vi "Main.vi"(10 "DAQ Type":enum16{"Hardware", "Simulation"}(ring), 11 "Module Admin":refnum<class "Delacor_lib_QMH_Module Admin.lvclass">) -> ()   [LabVIEW 2021, in "DC PWS.lvlib"]
doc: "This template is based off of the Queued Message Handler design pattern and the Queued Message Handler project template that ships with LabVIEW.\n\nThe main difference is that the queue is private to this module and communication between modules is performed via Broadcast and Request events.\n\nRequest events are wrapped in public API methods and are handled in the Event Handling Loop (EHL) of this VI. Any module can register for Broadcast events sent by this module. The EHL generates messages based on user interface actions.\n\nThe Message Handling Loop (MHL) processes messages generated by the EHL, or by other messages. The messages are string values, so new messages can be added easily to the Message Cases case structure in the MHL. Each message cluster can also provide an optional value for Message Data, which is a variant that can be converted to whatever message-specific data is required.\n_____\nBased on DQMH Project Template 6.1.0.94."
uses:
  DC PWS.lvlib
  <vilib>/Delacor/Delacor QMH/Libraries/Module Admin_class/Delacor_lib_QMH_Module Admin.lvclass
  Class/BK-Precision/BK-Precision.lvclass
  C:/repository/common_ATE/Libraries/DC PWS/Class/Abstract/Abstract.lvclass
  Class/Abstract/Abstract.lvclass
  Module Data--cluster.ctl
  <vilib>/Delacor/Delacor QMH/Libraries/Message Queue_class/Delacor_lib_QMH_Message Queue.lvclass/Delacor_lib_QMH_Message Queue.ctl
  Stop Argument--cluster.ctl
  <vilib>/Delacor/Delacor QMH/Libraries/Module Admin_class/Delacor_lib_QMH_Module Admin.lvclass/Delacor_lib_QMH_Module Admin.ctl
  REQ Initialize Hardware Argument--cluster.ctl
  REQ Initialize Hardware (Reply Payload)--cluster.ctl
  REQ Config Current Limit Argument--cluster.ctl
  REQ Over Voltage Limit Argument--cluster.ctl
  REQ Configure Output Argument--cluster.ctl
  REQ Enable Output Argument--cluster.ctl
  REQ Measurement Argument--cluster.ctl
  REQ Measurement (Reply Payload)--cluster.ctl
  REQ Close Ref Argument--cluster.ctl
  <vilib>/Utility/miscctls.llb/LVPointTypeDef.ctl
  <vilib>/Delacor/Delacor QMH/Libraries/Message Queue_class/Delacor_lib_QMH_Enqueue Message (Single).vi
  <vilib>/Delacor/Delacor QMH/Libraries/Module Admin_class/Delacor_lib_QMH_Get External Launch.vi
  <vilib>/Utility/error.llb/Error Cluster From Error Code.vi
  <vilib>/ErrorRing/Error Ring.xnode
  <vilib>/Delacor/Delacor QMH/Libraries/Message Queue_class/Delacor_lib_QMH_Message Queue.lvclass
panel:
  out "error out":errorcluster
  out "Status":string
  in  "Simulate MHL Error":bool
  in  "Simulate EHL Error":bool
  # "Other QMH Modules communicate with this Module via its Public API (wrappers for its Request Events).\n\nThis Module communicates with other Modules via its Broadcast Events.\nAny module that wants to get these messages, just registers for this module's Broadcast events."
  # "This template is for the Delacor Modified Queued Message Handler design pattern.\n\nSee the block diagram for more information on how to use this template."
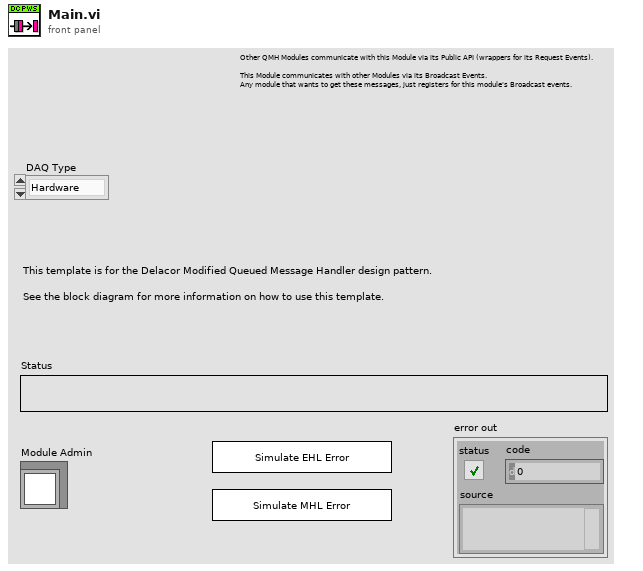
[diagram p1: front panel]
types:
  T1 = typedef "DC PWS.lvlib/Request Events--cluster.ctl" = cluster{"Stop Module":refnum<user-event>, "Show Panel":refnum<user-event>, "Hide Panel":refnum<user-event>, "Get Module Execution Status":refnum<user-event>, "Show Diagram":refnum<user-event>, "REQ Initialize Hardware":refnum<user-event>, "REQ Config Current Limit":refnum<user-event>, "REQ Over Voltage Limit":refnum<user-event>, "REQ Configure Output":refnum<user-event>, "REQ Enable Output":refnum<user-event>, "REQ Measurement":refnum<user-event>, "REQ Close Ref":refnum<user-event>}
  T2 = typedef "DC PWS.lvlib/Module Data--cluster.ctl" = cluster{"Status":string, "Abstract.lvclass":refnum<class "Abstract.lvclass">, "Connection Setting":cluster{"Connection Ref":variant, "Serial Configuration":cluster{"Baud Rate":u32}}}
  T3 = enum32{"invalid lock state", "Not Locked", "Locked (No Password)", "Password-protected"}
  T4 = typedef "DC PWS.lvlib/Stop Argument--cluster.ctl" = cluster{"Origin":string, "Exit via Stop Module Req?":bool, "Wait for Module to stop?":bool}
  T5 = typedef "DC PWS.lvlib/REQ Initialize Hardware Argument--cluster.ctl" = cluster{"Connection Setting":cluster{"Connection Ref":variant, "Serial Configuration":cluster{"Baud Rate":u32}}, "Wait Notifier":refnum<notifier>, "wait for reply":bool}
  T6 = typedef "DC PWS.lvlib/REQ Config Current Limit Argument--cluster.ctl" = cluster{"Current Limit Setting":cluster{"Address":dbl, "Current Limit":dbl}}
  T7 = typedef "DC PWS.lvlib/REQ Over Voltage Limit Argument--cluster.ctl" = cluster{"Over Voltage Setting":cluster{"Address":dbl, "Over Voltage Limit":dbl, "Protection Delay":dbl}}
  T8 = typedef "DC PWS.lvlib/REQ Configure Output Argument--cluster.ctl" = cluster{"Output Setting":cluster{"Address":dbl, "Voltage Level":dbl, "Enable Output":bool}}
  T9 = typedef "DC PWS.lvlib/REQ Enable Output Argument--cluster.ctl" = cluster{"Cluster":cluster{"Address":dbl, "Ouput":bool}}
  T10 = typedef "DC PWS.lvlib/REQ Measurement Argument--cluster.ctl" = cluster{"Wait Notifier":refnum<notifier>, "wait for reply":bool, "Meas Parameter":cluster{"Meas Command":enum16{"Voltage", "Current", "Power"}, "Address":dbl}}
  T11 = typedef "DC PWS.lvlib/REQ Close Ref Argument--cluster.ctl" = cluster{"Boolean":bool}
  T12 = typedef "LVPointTypeDef.ctl" = cluster{"Horizontal":i16, "Vertical":i16}
  T13 = enum32{"Invalid", "Standard", "Closed", "Hidden", "Minimized", "Maximized"}
  T14 = typedef "DC PWS.lvlib/REQ Initialize Hardware (Reply Payload)--cluster.ctl" = cluster{"Connect?":bool, "error":errorcluster}
  T15 = typedef "DC PWS.lvlib/REQ Measurement (Reply Payload)--cluster.ctl" = cluster{"error":errorcluster, "Value":dbl}
  T16 = cluster{"Connection Ref":variant, "Serial Configuration":cluster{"Baud Rate":u32}}
  T17 = cluster{"Address":dbl, "Over Voltage Limit":dbl, "Protection Delay":dbl}
  T18 = cluster{"Address":dbl, "Voltage Level":dbl, "Enable Output":bool}
  T19 = cluster{"Meas Command":enum16{"Voltage", "Current", "Power"}, "Address":dbl}
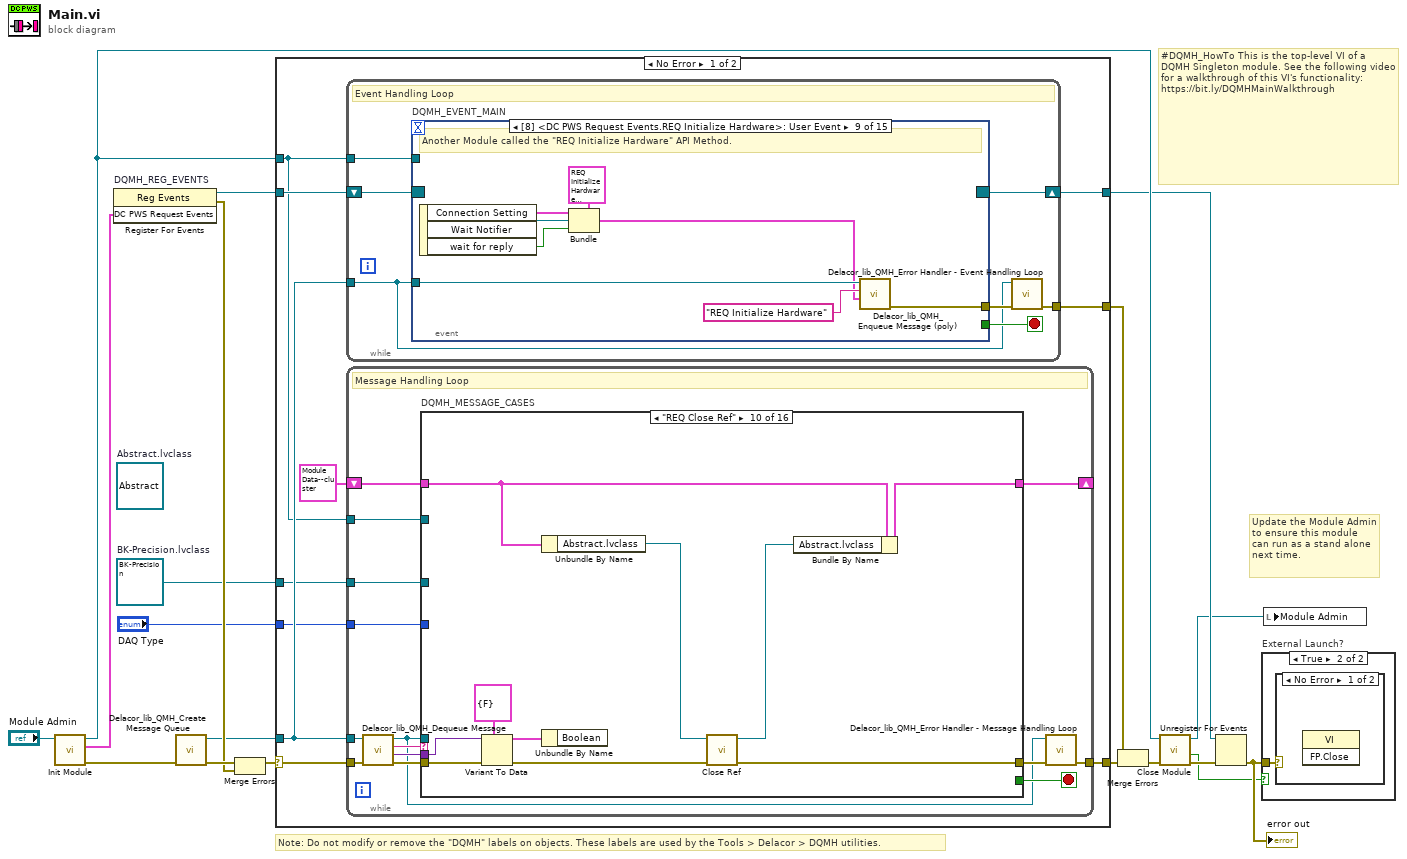
[diagram p0: block diagram]
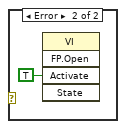
[diagram p3: hidden frame]
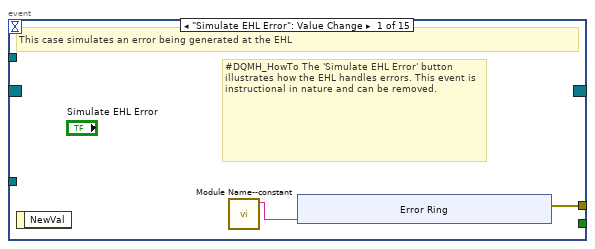
[diagram p4: hidden frame]
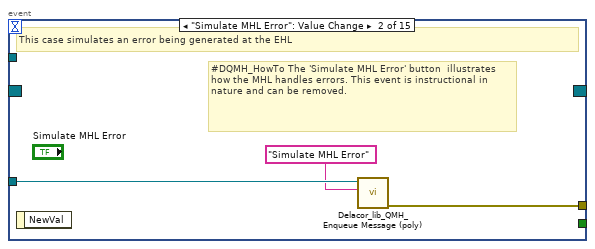
[diagram p5: hidden frame]
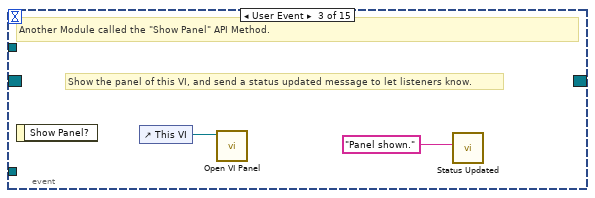
[diagram p6: hidden frame]
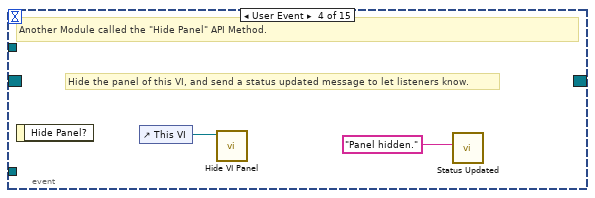
[diagram p7: hidden frame]
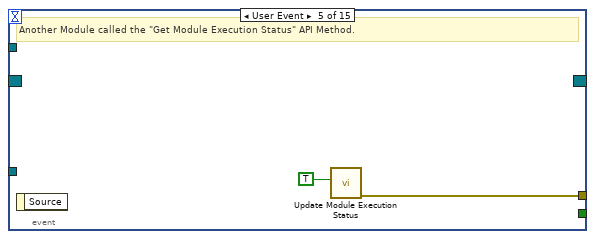
[diagram p8: hidden frame]
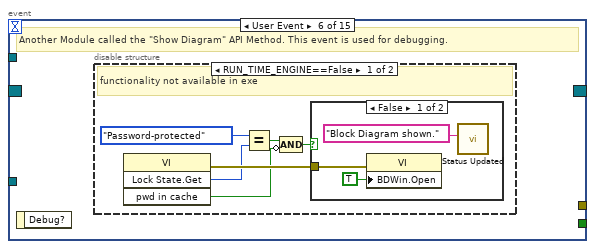
[diagram p9: hidden frame]
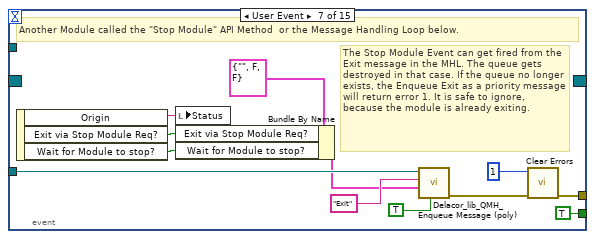
[diagram p12: hidden frame]
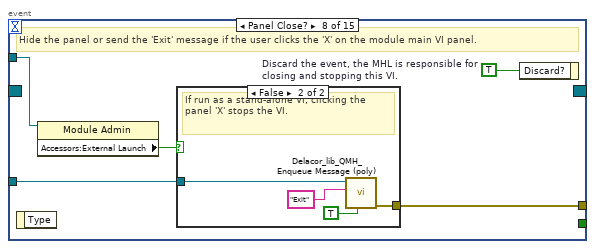
[diagram p13: hidden frame]
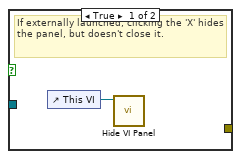
[diagram p14: hidden frame]
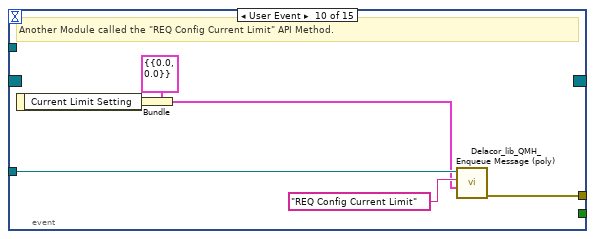
[diagram p15: hidden frame]
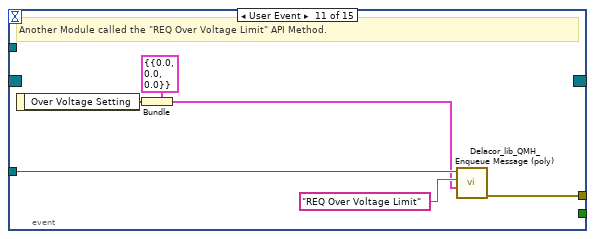
[diagram p16: hidden frame]
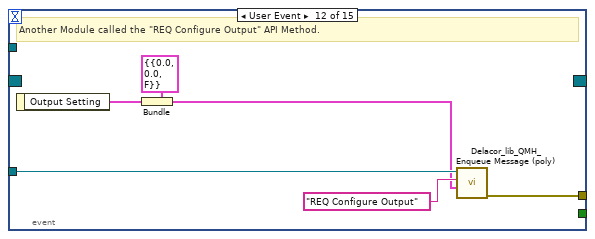
[diagram p17: hidden frame]
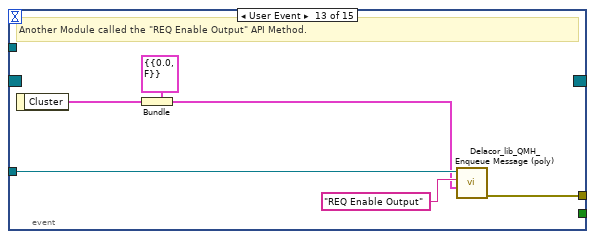
[diagram p18: hidden frame]
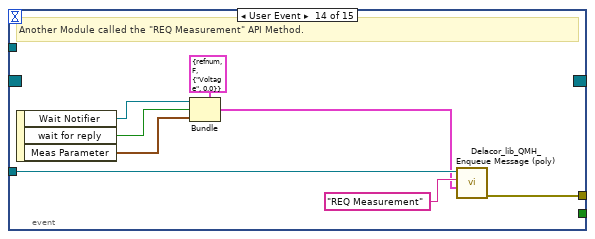
[diagram p19: hidden frame]
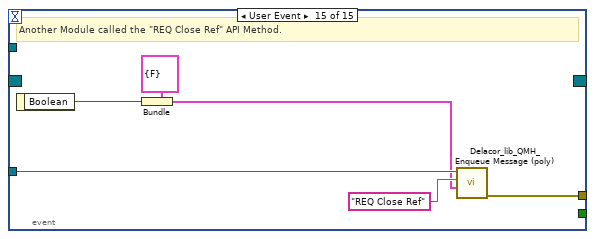
[diagram p20: hidden frame]
diagram:
  w2 = refnum<class "BK-Precision.lvclass"> refnum  # BK-Precision.lvclass
  (unwired) refnum<class "Abstract.lvclass"> refnum  # Abstract.lvclass
  # "#DQMH_HowTo This is the top-level VI of a DQMH Singleton module. See the following video for a walkthrough of this VI's functionality: https://bit.ly/DQMHMainWalkthrough"
  # "Note: Do not modify or remove the \"DQMH\" labels on objects. These labels are used by the Tools > Delacor > DQMH utilities."
  # "Update the Module Admin to ensure this module can run as a stand alone next time."
  n1 = call "Init Module.vi"("Singleton Module Admin in"="Module Admin") -> ("error out"=w18:errorcluster, "DC PWS Request Events"=w7:T1, "Singleton Module Admin out"=w10:refnum<class "Delacor_lib_QMH_Module Admin.lvclass">)  [unwired: 8 in]
  n2 = register-events "DQMH_REG_EVENTS"(w7) -> (reference out=w8:refnum<event-registration>, error out=w11:errorcluster)  [unwired: 2 in]
  n3 = call <vilib>:"Delacor_lib_QMH_Create Message Queue.vi"("error in"=w18) -> ("error out"=w13:errorcluster, "Message Queue"=w6:refnum<class "Delacor_lib_QMH_Message Queue.lvclass">)  [unwired: 9 in]
  n4 = Merge Errors(w13, w11) -> (w12:errorcluster)
  n5 = case shown="No Error" w12 {
    selector: w12 -> [w27 w339]
    tunnel: [w29 w338] -> w19
    tunnel: [w26 w344] -> w9
    tunnel: w8 -> [w24 w344]
    tunnel: w6 -> [w23 w337]
    tunnel: [w28 _] -> w16
    tunnel: w10 -> [w22 w340]
    tunnel: w2 -> [w21 _]
    tunnel: "DAQ Type" -> [w20 _]
    frame No Error {
      n6 = while {
        tunnel: w23 -> [w30]
        shift-right: [w33] -> w26
        shift-left: w24 -> [w34]
        tunnel: [w35] -> w28
        tunnel: w22 -> [w31]
        stop <- w32 stop-if-true
        # "Event Handling Loop"
        n7 = event "DQMH_EVENT_MAIN" shown="[8] <DC PWS Request Events.REQ Initialize Hardware>: User Event" {
          selector: w34 -> [_ _ _ _ _ _ _ _ _ _ _ _ _ _ _]
          dyn-events: [_ _ _ _ _ _ _ _ _ _ _ _ _ _ _] -> w33
          timeout: _ -> [_ _ _ _ _ _ _ _ _ _ _ _ _ _ _]
          tunnel: [_ _ _ _ _ _ TRUE ("Discard?") _ _ _ _ _ _ _ _] -> w32
          tunnel: w30 -> [_ w47 _ _ _ _ w71 w78 w93 w99 w105 w111 w117 w125 w131]
          tunnel: [w38 w48 _ _ w54 _ w74 w80 w86 w94 w100 w106 w112 w121 w126] -> w36
          tunnel: w31 -> [_ _ _ _ _ _ _ w77 _ _ _ _ _ _ _]
          event "Simulate EHL Error": Value Change {
            # "#DQMH_HowTo The 'Simulate EHL Error' button  illustrates how the EHL handles errors. This event is instructional in nature and can be removed."
            # "This case simulates an error being generated at the EHL"
            n8 = event-data() -> ()  [unwired: 1 in, 1 out]
            n9 = call "Module Name--constant.vi"() -> ("Module Name"=w37:string)  [unwired: 11 in]
            n10 = xnode "Error Ring"("parameter 0"=w37) -> ("error out"=w38:errorcluster)
          }
          event "Simulate MHL Error": Value Change {
            # "#DQMH_HowTo The 'Simulate MHL Error' button  illustrates how the MHL handles errors. This event is instructional in nature and can be removed."
            # "This case simulates an error being generated at the EHL"
            n11 = event-data() -> ()  [unwired: 1 in, 1 out]
            n12 = call-poly <vilib>:"Delacor_lib_QMH_Enqueue Message (poly).vi"("Message"="Simulate MHL Error", "Message Queue in"=w47) -> ("error out"=w48:errorcluster)  [unwired: 8 in, 1 out]
          }
          event User Event {
            # "Show the panel of this VI, and send a status updated message to let listeners know."
            # "Another Module called the \"Show Panel\" API Method."
            n13 = event-data() -> ()  [unwired: 1 in, 1 out]
            n14 = control-ref of="This VI"() -> (w50:refnum<vi>)
            n15 = call "Open VI Panel.vi"("VI"=w50) -> ()  [unwired: 10 in, 1 out]
            n16 = call "Status Updated.vi"("Status"="Panel shown." ("format string")) -> ()  [unwired: 10 in, 1 out]
          }
          event User Event {
            # "Hide the panel of this VI, and send a status updated message to let listeners know."
            # "Another Module called the \"Hide Panel\" API Method."
            n17 = event-data() -> ()  [unwired: 1 in, 1 out]
            n18 = control-ref of="This VI"() -> (w52:refnum<vi>)
            n19 = call "Hide VI Panel.vi"("VI"=w52) -> ()  [unwired: 10 in, 1 out]
            n20 = call "Status Updated.vi"("Status"="Panel hidden." ("format string")) -> ()  [unwired: 10 in, 1 out]
          }
          event User Event {
            # "Another Module called the \"Get Module Execution Status\" API Method."
            n21 = event-data() -> ()  [unwired: 1 in, 1 out]
            n22 = call "Update Module Execution Status.vi"("Running?"=TRUE) -> ("error out"=w54:errorcluster)  [unwired: 10 in]
          }
          event User Event {
            # "Another Module called the \"Show Diagram\" API Method. This event is used for debugging."
            n23 = event-data() -> ()  [unwired: 1 in, 1 out]
            n24 = disable-structure shown="RUN_TIME_ENGINE==False" {
              frame condition #0 (active) {
                # "functionality not available in exe"
                n25 = invoke class="VI" method="Lock State.Get"() -> (error out=w60:errorcluster, "Get Lock State"=w59:T3, "pwd in cache"=w56:bool)  [unwired: 4 in, 1 out]
                n26 = Equal?(x=T3."Password-protected", y=w59) -> (x = y?=w57:bool)
                n27 = Compound Arithmetic op=AND(w57, invert w56) -> (w55:bool)
                n28 = case shown="False" w55 {
                  tunnel: w60 -> [w63 _]
                  frame False {
                    n29 = property class="VI"(error in=w63, "BDWin.Open"=TRUE ("Block Diagram Window:Open")) -> ()  [unwired: 1 in, 2 out]
                    n30 = call "Status Updated.vi"("Status"="Block Diagram shown." ("format string")) -> ()  [unwired: 10 in, 1 out]
                  }
                  frame True {
                    # "Password-protected VI, and the password is not in the cache. Do not show the diagram."
                  }
                }
              }
              frame condition #1 {
              }
            }
          }
          event User Event {
            # "The Stop Module Event can get fired from the Exit message in the MHL. The queue gets destroyed in that case. If the queue no longer exists, the Enqueue Exit as a priority message will return error 1. It is safe to ignore, because the module is already exiting."
            # "Another Module called the \"Stop Module\" API Method  or the Message Handling Loop below."
            n31 = event-data() -> ("Origin"=w70:string, "Exit via Stop Module Req?"=w66:bool, "Wait for Module to stop?"=w65:bool)  [unwired: 1 in]
            n32 = local write "Status"(w70) -> ()
            n33 = Bundle By Name(cluster=T4 {"Origin"="", "Exit via Stop Module Req?"=FALSE, "Wait for Module to stop?"=FALSE} ("Stop Argument"), "Exit via Stop Module Req?"=w66, "Wait for Module to stop?"=w65) -> (w64:T4)
            n34 = call-poly <vilib>:"Delacor_lib_QMH_Enqueue Message (poly).vi"("Priority Message? (F)"=TRUE, "Message Data"=w64, "Message"="Exit", "Message Queue in"=w71) -> ("error out"=w75:errorcluster)  [unwired: 6 in, 1 out]
            n35 = call <vilib>:"Clear Errors.vi"("error in (no error)"=w75, "specific error code to clear (0: all)"=1) -> ("error out"=w74:errorcluster)  [unwired: 4 in, 1 out]
          }
          event Panel Close? {
            w79 = TRUE  # Discard the event, the MHL is responsible for closing and stopping this VI.
            # "Hide the panel or send the 'Exit' message if the user clicks the 'X' on the module main VI panel."
            n36 = event-data() -> ()  [unwired: 1 in, 1 out]
            n37 = property class="Module Admin"(reference=w77) -> ("Accessors:External Launch"=w76:bool)  [unwired: 1 in, 2 out]
            n38 = case shown="False" w76 {
              tunnel: w78 -> [_ w84]
              tunnel: [_ w85] -> w80
              frame True {
                # "If externally launched, clicking the 'X' hides the panel, but doesn't close it."
                n39 = control-ref of="This VI"() -> (w81:refnum<vi>)
                n40 = call "Hide VI Panel.vi"("VI"=w81) -> ()  [unwired: 10 in, 1 out]
              }
              frame False {
                # "If run as a stand-alone VI, clicking the panel 'X' stops the VI."
                n41 = call-poly <vilib>:"Delacor_lib_QMH_Enqueue Message (poly).vi"("Priority Message? (F)"=TRUE, "Message"="Exit", "Message Queue in"=w84) -> ("error out"=w85:errorcluster)  [unwired: 7 in, 1 out]
              }
            }
            n42 = event-data("Discard?"=w79) -> ()  [unwired: 1 in, 1 out]
          }
          event User Event {
            # "Another Module called the \"REQ Initialize Hardware\" API Method."
            n43 = event-data() -> ("Connection Setting"=w89:T16, "Wait Notifier"=w88:refnum<notifier>, "wait for reply"=w87:bool)  [unwired: 1 in]
            n44 = Bundle(cluster=T5 {"Connection Setting"={"Connection Ref"=variant, "Serial Configuration"={"Baud Rate"=9600}}, "Wait Notifier"=refnum, "wait for reply"=FALSE} ("REQ Initialize Hardware Argument"), "Connection Setting"=w89, "Wait Notifier"=w88, "wait for reply"=w87) -> (w90:T5)
            n45 = call-poly <vilib>:"Delacor_lib_QMH_Enqueue Message (poly).vi"("Message Data"=w90, "Message"="REQ Initialize Hardware", "Message Queue in"=w93) -> ("error out"=w86:errorcluster)  [unwired: 7 in, 1 out]
          }
          event User Event {
            # "Another Module called the \"REQ Config Current Limit\" API Method."
            n46 = event-data() -> ("Current Limit Setting"=w95:cluster{"Address":dbl, "Current Limit":dbl})  [unwired: 1 in]
            n47 = Bundle(cluster=T6 {"Current Limit Setting"={"Address"=0.0, "Current Limit"=0.0}} ("REQ Config Current Limit Argument"), "Current Limit Setting"=w95) -> (w96:T6)
            n48 = call-poly <vilib>:"Delacor_lib_QMH_Enqueue Message (poly).vi"("Message Data"=w96, "Message"="REQ Config Current Limit", "Message Queue in"=w99) -> ("error out"=w94:errorcluster)  [unwired: 7 in, 1 out]
          }
          event User Event {
            # "Another Module called the \"REQ Over Voltage Limit\" API Method."
            n49 = event-data() -> ("Over Voltage Setting"=w101:T17)  [unwired: 1 in]
            n50 = Bundle(cluster=T7 {"Over Voltage Setting"={"Address"=0.0, "Over Voltage Limit"=0.0, "Protection Delay"=0.0}} ("REQ Over Voltage Limit Argument"), "Over Voltage Setting"=w101) -> (w102:T7)
            n51 = call-poly <vilib>:"Delacor_lib_QMH_Enqueue Message (poly).vi"("Message Data"=w102, "Message"="REQ Over Voltage Limit", "Message Queue in"=w105) -> ("error out"=w100:errorcluster)  [unwired: 7 in, 1 out]
          }
          event User Event {
            # "Another Module called the \"REQ Configure Output\" API Method."
            n52 = event-data() -> ("Output Setting"=w107:T18)  [unwired: 1 in]
            n53 = Bundle(cluster=T8 {"Output Setting"={"Address"=0.0, "Voltage Level"=0.0, "Enable Output"=FALSE}} ("REQ Configure Output Argument"), "Output Setting"=w107) -> (w108:T8)
            n54 = call-poly <vilib>:"Delacor_lib_QMH_Enqueue Message (poly).vi"("Message Data"=w108, "Message"="REQ Configure Output", "Message Queue in"=w111) -> ("error out"=w106:errorcluster)  [unwired: 7 in, 1 out]
          }
          event User Event {
            # "Another Module called the \"REQ Enable Output\" API Method."
            n55 = event-data() -> ("Cluster"=w113:cluster{"Address":dbl, "Ouput":bool})  [unwired: 1 in]
            n56 = Bundle(cluster=T9 {"Cluster"={"Address"=0.0, "Ouput"=FALSE}} ("REQ Enable Output Argument"), "Cluster"=w113) -> (w114:T9)
            n57 = call-poly <vilib>:"Delacor_lib_QMH_Enqueue Message (poly).vi"("Message Data"=w114, "Message"="REQ Enable Output", "Message Queue in"=w117) -> ("error out"=w112:errorcluster)  [unwired: 7 in, 1 out]
          }
          event User Event {
            # "Another Module called the \"REQ Measurement\" API Method."
            n58 = event-data() -> ("Wait Notifier"=w120:refnum<notifier>, "wait for reply"=w119:bool, "Meas Parameter"=w118:T19)  [unwired: 1 in]
            n59 = Bundle(cluster=T10 {"Wait Notifier"=refnum, "wait for reply"=FALSE, "Meas Parameter"={"Meas Command"=enum."Voltage", "Address"=0.0}} ("REQ Measurement Argument"), "Wait Notifier"=w120, "wait for reply"=w119, "Meas Parameter"=w118) -> (w122:T10)
            n60 = call-poly <vilib>:"Delacor_lib_QMH_Enqueue Message (poly).vi"("Message Data"=w122, "Message"="REQ Measurement", "Message Queue in"=w125) -> ("error out"=w121:errorcluster)  [unwired: 7 in, 1 out]
          }
          event User Event {
            # "Another Module called the \"REQ Close Ref\" API Method."
            n61 = event-data() -> ("Boolean"=w127:bool)  [unwired: 1 in]
            n62 = Bundle(cluster=T11 {"Boolean"=FALSE} ("REQ Close Ref Argument"), "Boolean"=w127) -> (w128:T11)
            n63 = call-poly <vilib>:"Delacor_lib_QMH_Enqueue Message (poly).vi"("Message Data"=w128, "Message"="REQ Close Ref", "Message Queue in"=w131) -> ("error out"=w126:errorcluster)  [unwired: 7 in, 1 out]
          }
        }
        n64 = call-dynamic "Delacor_lib_QMH_Error Handler - Event Handling Loop.vi"("error in"=w36, "Message Queue in"=w30) -> ("dup error in"=w35:errorcluster)  [unwired: 8 in, 1 out]
      }
      n65 = while {
        tunnel: w23 -> [w136]
        shift-right: [w140] -> _
        shift-left: T2 {"Status"="", "Abstract.lvclass"=refnum, "Connection Setting"={"Connection Ref"=variant, "Serial Configuration"={"Baud Rate"=9600}}} ("Data Cluster") -> [w141]
        tunnel: w27 -> [w144]
        tunnel: [w142] -> w29
        tunnel: w22 -> [w134]
        tunnel: w21 -> [w133]
        tunnel: w20 -> [w132]
        stop <- w139 stop-if-true
        # "Message Handling Loop"
        n66 = call-dynamic "Delacor_lib_QMH_Dequeue Message.vi"("error in"=w144, "Message Queue in"=w136) -> ("error out"=w143:errorcluster, "Message Data"=w137:variant, "Message"=w138:string, "Message Queue out"=w135:refnum<class "Delacor_lib_QMH_Message Queue.lvclass">)  [unwired: 6 in]
        n67 = case "DQMH_MESSAGE_CASES" shown="\"REQ Close Ref\"" w138 {
          selector: w138 -> [_ _ _ _ _ _ _ _ _ _ _ _ _ _ _ w324]
          tunnel: w135 -> [_ _ _ _ _ _ _ _ w255 _ _ _ _ w289 w320 _]
          tunnel: w143 -> [w164 w168 w186 w199 w210 w221 w232 w248 w257 w269 w272 w274 w279 w296 w322 w326]
          tunnel: [w162 w168 w175 w194 w200 w216 w222 w234 w256 w264 w271 w274 w278 w292 w304 w327] -> w145
          tunnel: w141 -> [w153 w167 w170 w192 w204 w214 w226 w238 w254 w263 w270 w273 w276 w291 w311 w325]
          tunnel: [w152 w167 w177 w190 w202 w212 w224 w236 w254 w261 w270 w273 w276 w291 w308 w325] -> w140
          tunnel: [_ _ _ _ _ _ _ _ _ _ _ _ _ _ w319 _] -> w139
          tunnel: w137 -> [_ _ w185 w198 w209 w220 w231 w247 _ w268 _ _ _ w290 w318 _]
          tunnel: w134 -> [w154 _ _ _ _ _ _ _ _ _ _ _ _ w288 w313 _]
          tunnel: w133 -> [w146 _ _ _ _ _ _ _ _ _ _ _ _ _ _ _]
          tunnel: w132 -> [_ _ w172 _ _ _ _ _ _ _ _ _ _ _ _ _]
          frame "Initialize" {
            w148 = "Initial Message" ("Initial Message")
            # "Initialize - Any operation that needs to be done before the module can receive messages. Synchronize Caller Events.vi will inform Start Module.vi that the module has launched and is ready to receive messages. Module Did Init.vi will broadcast that the module initialized."
            n68 = call "Synchronize Caller Events.vi"("error in (no error)"=w164, "Singleton Module Admin in"=w154) -> ("error out"=w163:errorcluster, "Singleton Module Admin out"=w149:refnum<class "Delacor_lib_QMH_Module Admin.lvclass">)  [unwired: 8 in]
            n69 = property class="Module Admin"(reference=w149) -> ("Accessors:External Launch"=w158:bool)  [unwired: 1 in, 2 out]
            n70 = Select(t=T13."Hidden" ("State"), s=w158, f=T13."Standard" ("State")) -> (s? t:f=w155:T13)
            n71 = call "Module Name--constant.vi"() -> ("Module Name"=w161:string)  [unwired: 11 in]
            n72 = Bundle By Name(cluster=w153, "Status"=w148, "Abstract.lvclass"=w146) -> (w152:T2)
            n73 = property class="VI"("Front Panel.Title"=w161) -> (reference out=w160:refnum<vi>, error out=w166:errorcluster)  [unwired: 2 in]
            n74 = call "Module Name--constant.vi"() -> ("Module Name"=w150:string)  [unwired: 11 in]
            n75 = invoke class="VI" method="FP.Open"(reference=w160, error in=w166, "State"=w155) -> (reference out=w159:refnum<vi>, error out=w165:errorcluster)  [unwired: 2 in, 3 out]
            n76 = call "Module Did Init.vi"("error in (no error)"=w163, "Initialized?"=TRUE, "Origin"=w150) -> ("error out"=w162:errorcluster)  [unwired: 8 in]
            n77 = invoke class="VI" method="FP.Center"(reference=w159, error in=w165) -> ()  [unwired: 1 in, 3 out]
            n78 = property on="Pane" class="Pane"("Origin"=T12 {"Horizontal"=0, "Vertical"=0}) -> ()  [unwired: 2 in, 2 out]
            "Status" <- w148
          }
          frame "---Module Specific---" {
            # "Separator -- The following cases handle messages specific to this Module."
          }
          frame "REQ Initialize Hardware" {
            n79 = Variant To Data(error in=w186, type=T5 {"Connection Setting"={"Connection Ref"=variant, "Serial Configuration"={"Baud Rate"=9600}}, "Wait Notifier"=refnum, "wait for reply"=FALSE} ("REQ Initialize Hardware Argument"), Variant=w185) -> (data=w183:T5, error out=w178:errorcluster)
            n80 = Unbundle By Name(w183) -> ("Wait Notifier"=w182:refnum<notifier>, "wait for reply"=w181:bool, "Connection Setting"=w171:T16)
            n81 = Unbundle By Name(w170) -> ("Abstract.lvclass"=w169:refnum<class "Abstract.lvclass">)
            n82 = call-dynamic "Initialize Hardware.vi"("error in (no error)"=w178, "Connection Setting"=w171, "DAQ Type"=w172, "Abstract in"=w169) -> ("error out"=w175:errorcluster, "Abstract out"=w176:refnum<class "Abstract.lvclass">)  [unwired: 6 in]
            n83 = Unbundle By Name(w175) -> ("status"=w174:bool)
            n84 = Bundle By Name(cluster=w170, "Connection Setting"=w171, "Abstract.lvclass"=w176) -> (w177:T2)
            n85 = Not(x=w174) -> (.not. x?=w173:bool)
            n86 = Bundle By Name(cluster=T14 {"Connect?"=FALSE, "error"={"status"=FALSE, "code"=0, "source"=""}} ("REQ Initialize Hardware (Reply Payload)"), "Connect?"=w173) -> (w180:T14)
            n87 = case shown="True" w181 {
              tunnel: w182 -> [_ w188]
              tunnel: w180 -> [_ w187]
              frame False {
              }
              frame True {
                n88 = Send Notification(notification=w187, notifier=w188) -> ()  [unwired: 1 in, 2 out]
              }
            }
          }
          frame "REQ Config Current Limit" {
            n89 = Variant To Data(error in=w199, type=T6 {"Current Limit Setting"={"Address"=0.0, "Current Limit"=0.0}} ("REQ Config Current Limit Argument"), Variant=w198) -> (data=w196:T6, error out=w195:errorcluster)
            n90 = Unbundle By Name(w196) -> ("Current Limit Setting"=w193:cluster{"Address":dbl, "Current Limit":dbl})
            n91 = Unbundle By Name(w192) -> ("Abstract.lvclass"=w191:refnum<class "Abstract.lvclass">)
            n92 = call-dynamic "Configure Current Limit.vi"("error in (no error)"=w195, "Current Limit Setting"=w193, "Abstract in"=w191) -> ("error out"=w194:errorcluster, "Abstract out"=w189:refnum<class "Abstract.lvclass">)  [unwired: 7 in]
            n93 = Bundle By Name(cluster=w192, "Abstract.lvclass"=w189) -> (w190:T2)
          }
          frame "REQ Over Voltage Limit" {
            n94 = Variant To Data(error in=w210, type=T7 {"Over Voltage Setting"={"Address"=0.0, "Over Voltage Limit"=0.0, "Protection Delay"=0.0}} ("REQ Over Voltage Limit Argument"), Variant=w209) -> (data=w207:T7, error out=w206:errorcluster)
            n95 = Unbundle By Name(w207) -> ("Over Voltage Setting"=w205:T17)
            n96 = Unbundle By Name(w204) -> ("Abstract.lvclass"=w203:refnum<class "Abstract.lvclass">)
            n97 = call-dynamic "Configure Over Voltage Limit.vi"("error in (no error)"=w206, "Over Voltage Setting"=w205, "Abstract in"=w203) -> ("error out"=w200:errorcluster, "Abstract out"=w201:refnum<class "Abstract.lvclass">)  [unwired: 7 in]
            n98 = Bundle By Name(cluster=w204, "Abstract.lvclass"=w201) -> (w202:T2)
          }
          frame "REQ Configure Output" {
            n99 = Variant To Data(error in=w221, type=T8 {"Output Setting"={"Address"=0.0, "Voltage Level"=0.0, "Enable Output"=FALSE}} ("REQ Configure Output Argument"), Variant=w220) -> (data=w218:T8, error out=w217:errorcluster)
            n100 = Unbundle By Name(w218) -> ("Output Setting"=w215:T18)
            n101 = Unbundle By Name(w214) -> ("Abstract.lvclass"=w213:refnum<class "Abstract.lvclass">)
            n102 = call-dynamic "Configure Output.vi"("error in (no error)"=w217, "Output Setting"=w215, "Abstract in"=w213) -> ("error out"=w216:errorcluster, "Abstract out"=w211:refnum<class "Abstract.lvclass">)  [unwired: 7 in]
            n103 = Bundle By Name(cluster=w214, "Abstract.lvclass"=w211) -> (w212:T2)
          }
          frame "REQ Enable Output" {
            n104 = Variant To Data(error in=w232, type=T9 {"Cluster"={"Address"=0.0, "Ouput"=FALSE}} ("REQ Enable Output Argument"), Variant=w231) -> (data=w229:T9, error out=w228:errorcluster)
            n105 = Unbundle By Name(w229) -> ("Cluster"=w227:cluster{"Address":dbl, "Ouput":bool})
            n106 = Unbundle By Name(w226) -> ("Abstract.lvclass"=w225:refnum<class "Abstract.lvclass">)
            n107 = call-dynamic "Enable Output.vi"("error in (no error)"=w228, "Cluster"=w227, "Abstract in"=w225) -> ("error out"=w222:errorcluster, "Abstract out"=w223:refnum<class "Abstract.lvclass">)  [unwired: 7 in]
            n108 = Bundle By Name(cluster=w226, "Abstract.lvclass"=w223) -> (w224:T2)
          }
          frame "REQ Measurement" {
            n109 = Variant To Data(error in=w248, type=T10 {"Wait Notifier"=refnum, "wait for reply"=FALSE, "Meas Parameter"={"Meas Command"=enum."Voltage", "Address"=0.0}} ("REQ Measurement Argument"), Variant=w247) -> (data=w245:T10, error out=w240:errorcluster)
            n110 = Unbundle By Name(w245) -> ("Wait Notifier"=w244:refnum<notifier>, "wait for reply"=w243:bool, "Meas Parameter"=w239:T19)
            n111 = Unbundle By Name(w238) -> ("Abstract.lvclass"=w237:refnum<class "Abstract.lvclass">)
            n112 = call-dynamic "Measurement Parameter.vi"("error in (no error)"=w240, "Meas Parameter"=w239, "Abstract in"=w237) -> ("error out"=w234:errorcluster, "Value"=w233:dbl, "Abstract out"=w235:refnum<class "Abstract.lvclass">)  [unwired: 6 in]
            n113 = Bundle By Name(cluster=w238, "Abstract.lvclass"=w235) -> (w236:T2)
            n114 = Bundle By Name(cluster=T15 {"error"={"status"=FALSE, "code"=0, "source"=""}, "Value"=0.0} ("REQ Measurement (Reply Payload)"), "Value"=w233) -> (w242:T15)
            n115 = case shown="True" w243 {
              tunnel: w244 -> [_ w250]
              tunnel: w242 -> [_ w249]
              frame False {
              }
              frame True {
                n116 = Send Notification(notification=w249, notifier=w250) -> ()  [unwired: 1 in, 2 out]
              }
            }
          }
          frame "REQ Reconnect" {
            # "Duplicate this frame when creating new messages.  Change this comment in the duplicated frame to describe this message."
            n117 = Unbundle By Name(w254) -> ("Connection Setting.Connection Ref"=w253:variant)
            n118 = Bundle By Name(cluster=T5 {"Connection Setting"={"Connection Ref"=variant, "Serial Configuration"={"Baud Rate"=9600}}, "Wait Notifier"=refnum, "wait for reply"=FALSE} ("REQ Initialize Hardware Argument"), "Connection Setting.Connection Ref"=w253) -> (w252:T5)
            n119 = Wait (ms)(milliseconds to wait=u32 1000) -> ()  [unwired: 1 out]
            n120 = call-poly <vilib>:"Delacor_lib_QMH_Enqueue Message (poly).vi"("error in"=w257, "Message Data"=w252, "Message"="REQ Initialize Hardware", "Message Queue in"=w255) -> ("error out"=w256:errorcluster)  [unwired: 6 in, 1 out]
          }
          frame "REQ Close Ref" {
            n121 = Variant To Data(error in=w269, type=T11 {"Boolean"=FALSE} ("REQ Close Ref Argument"), Variant=w268) -> (data=w266:T11, error out=w265:errorcluster)
            n122 = Unbundle By Name(w263) -> ("Abstract.lvclass"=w262:refnum<class "Abstract.lvclass">)
            n123 = Unbundle By Name(w266) -> ()  [unwired: 1 out]
            n124 = call-dynamic "Close Ref.vi"("error in (no error)"=w265, "Abstract in"=w262) -> ("error out"=w264:errorcluster, "Abstract out"=w260:refnum<class "Abstract.lvclass">)  [unwired: 8 in]
            n125 = Bundle By Name(cluster=w263, "Abstract.lvclass"=w260) -> (w261:T2)
          }
          frame "---Copy This Frame---" {
            # "Duplicate this frame when creating new messages.  Change this comment in the duplicated frame to describe this message."
            n126 = Merge Errors(w272) -> (w271:errorcluster)
          }
          frame "---Exit and Error Handling---" {
            # "Separator - The following cases handle errors and exit messages."
          }
          frame "Simulate MHL Error" {
            # "#DQMH_HowTo The 'Simulate MHL Error' button  illustrates how the MHL handles errors. This event is instructional in nature and can be removed."
            # "Simulate an error occurring at the MHL"
            n127 = call "Module Name--constant.vi"() -> ("Module Name"=w275:string)  [unwired: 11 in]
            n128 = xnode "Error Ring"("parameter 0"=w275) -> ("error out"=w277:errorcluster)
            n129 = Merge Errors(w279, w277) -> (w278:errorcluster)
          }
          frame "Error" {
            # "#CodeRecommended - If you ever change the name of this \"Error\" message, you'll need to update the name in the Check Loop Error.vi as well."
            # "#CodeRecommended - If the module is running in standalone mode (External Launch = FALSE), this code will pop up an error dialog and call the 'Exit' message if an error occurs. Add more fine-grained error handling here."
            # "Error - Check the error message data and respond accordingly. This message is sent by the \"Error Handler\" VIs at the end of each loop in this application."
            n130 = property class="Module Admin"(reference=w288) -> ("Accessors:External Launch"=w287:bool)  [unwired: 1 in, 2 out]
            n131 = Variant To Data(error in=w296, type=errorcluster {"status"=FALSE, "code"=0, "source"=""} ("error constant"), Variant=w290) -> (data=w297:errorcluster, error out=w294:errorcluster)
            n132 = call "Error Reported.vi"("Error"=w297) -> ()  [unwired: 10 in, 1 out]
            n133 = case shown="False" w287 {
              tunnel: [w302 _] -> w293
              tunnel: w289 -> [w300 _]
              tunnel: w297 -> [w301 _]
              frame False {
                n134 = call <vilib>:"Simple Error Handler.vi"("error in (no error)"=w301) -> ()  [unwired: 4 in, 5 out]
                n135 = call-poly <vilib>:"Delacor_lib_QMH_Enqueue Message (poly).vi"("Priority Message? (F)"=TRUE, "Message"="REQ Reconnect", "Message Queue in"=w300) -> ("error out"=w302:errorcluster)  [unwired: 7 in, 1 out]
              }
              frame True {
                # "If the module was launched externally, calling the Error Reported broadcast VI is the only action performed by the \"Error\" message. The module's caller can then process the error appropriately."
              }
            }
            n136 = Merge Errors(w294, w293) -> (w292:errorcluster)
            n137 = local write "error out"(w292) -> ()
          }
          frame "Exit" {
            w317 = 91  # 91: not all Exit messages will have an argument
            w319 = TRUE  # Stop the VI
            # "Release the message queue reference"
            # "Exit - Exit the application."
            n138 = Variant To Data(error in=w322, type=T4 {"Origin"="", "Exit via Stop Module Req?"=FALSE, "Wait for Module to stop?"=FALSE} ("Stop Argument"), Variant=w318) -> (data=w315:T4, error out=w321:errorcluster)
            n139 = control-ref of="This VI"() -> (w314:refnum<vi>)
            n140 = call <vilib>:"Clear Errors.vi"("error in (no error)"=w321, "specific error code to clear (0: all)"=w317) -> ("error out"=w312:errorcluster)  [unwired: 4 in, 1 out]
            n141 = Unbundle By Name(w311) -> ("Abstract.lvclass"=w310:refnum<class "Abstract.lvclass">)
            n142 = call "Handle Exit.vi"("Stop Argument"=w315, "Admin in"=w313, "VI reference"=w314) -> ("error out"=w309:errorcluster)  [unwired: 7 in, 1 out]
            n143 = call-dynamic "Close Ref.vi"("error in (no error)"=w309, "Abstract in"=w310) -> ("error out"=w305:errorcluster, "Abstract out"=w307:refnum<class "Abstract.lvclass">)  [unwired: 8 in]
            n144 = Bundle By Name(cluster=w311, "Abstract.lvclass"=w307) -> (w308:T2)
            n145 = call <vilib>:"Clear Errors.vi"("error in (no error)"=w305) -> ("error out"=w303:errorcluster)  [unwired: 5 in, 1 out]
            n146 = call-dynamic "Delacor_lib_QMH_Release Message Queue.vi"("error in"=w312, "Message Queue"=w320) -> ("error out"=w306:errorcluster)  [unwired: 9 in]
            n147 = Merge Errors(w303, w306) -> (w304:errorcluster)
          }
          frame Default {
            # "'Default' case only runs if there is a message that isn't defined in any of the other cases.  Output a programming error."
            n148 = call "Module Name--constant.vi"() -> ("Module Name"=w323:string)  [unwired: 11 in]
            n149 = xnode "Error Ring"("parameter 0"=w324, "parameter 1"=w323) -> ("error out"=w328:errorcluster)
            n150 = Merge Errors(w326, w328) -> (w327:errorcluster)
          }
        }
        n151 = call-dynamic "Delacor_lib_QMH_Error Handler - Message Handling Loop.vi"("error in"=w145, "Message Queue in"=w135) -> ("dup error in"=w142:errorcluster)  [unwired: 8 in, 1 out]
      }
    }
    frame Error {
      # "Synchronize Caller Events.vi will inform Start Module.vi that the module has launched and will let the code calling Start Module.vi register for broadcasts and would permit the caller receive the broadcast that an error occurred at launch time."
      n152 = call-dynamic "Delacor_lib_QMH_Release Message Queue.vi"("error in"=w339, "Message Queue"=w337) -> ("error out"=w338:errorcluster)  [unwired: 9 in]
      n153 = call "Synchronize Caller Events.vi"("Singleton Module Admin in"=w340) -> ("error out"=w345:errorcluster)  [unwired: 9 in, 1 out]
      n154 = call "Module Name--constant.vi"() -> ("Module Name"=w343:string)  [unwired: 11 in]
      n155 = Format Into String(format string="An error occurred during initialization. %s is no longer running.", w343) -> (resulting string=w341:string)  [unwired: 2 in, 1 out]
      n156 = Merge Errors(w338, w345) -> (w346:errorcluster)
      n157 = call "Error Reported.vi"("Additional Information"=w341, "Error"=w346) -> ()  [unwired: 9 in, 1 out]
    }
  }
  n158 = Merge Errors(w16, w19) -> (w15:errorcluster)
  n159 = call "Close Module.vi"("error in (no error)"=w15, "Module Admin in"=w10) -> ("error out"=w17:errorcluster, "External Launch"=w3:bool, "Module Admin out"=w4:refnum<class "Delacor_lib_QMH_Module Admin.lvclass">)  [unwired: 7 in]
  n160 = Unregister For Events(event registration refnum=w9, error in=w17) -> (error out=w14:errorcluster)
  "error out" <- w14
  n161 = case "External Launch?" shown="True" w3 {
    tunnel: w14 -> [_ w347]
    frame False {
    }
    frame True {
      n162 = case shown="No Error" w347 {
        frame No Error {
          n163 = invoke class="VI" method="FP.Close"() -> ()  [unwired: 3 in, 3 out]
        }
        frame Error {
          n164 = invoke class="VI" method="FP.Open"("Activate"=TRUE ("Activate?")) -> ()  [unwired: 4 in, 5 out]
        }
      }
    }
  }
  n165 = local write "Module Admin"(w4) -> ()
